vi "HostCoordinateCalibration.vi"(0 "stop_sign_queue":refnum<queue>, 4 "RetRate um/s":dbl format="%#_13g", 5 "AppRate um/s":dbl format="%#_13g", 6 "Retract um":dbl format="%#_13g", 7 "Threshold %":dbl format="%#_13g", 8 "YCalibrationEnd um":dbl format="%#_13g", 9 "XCalibrationEnd um":dbl format="%#_13g", 10 "YCalibrationOffset um":dbl format="%#_13g", 11 "XCalibrationOffset um":dbl format="%#_13g") -> (3 "img_bundle":i32[][][](array[numeric]))   [LabVIEW 2024]
uses:
  <vilib>/FPGAPlugInAG/USB-7845R OEM/niLvFpga_Open_USB-7845R OEM.vi
  <vilib>/rvi/interface/common/dynamic/niFpgaDynamicAddResources.vi
  <vilib>/Utility/error.llb/Error Cluster From Error Code.vi
  <vilib>/rvi/errors/niLvFpgaAdjustHostInterfaceError.vi
  <vilib>/FPGAPlugInAG/Dynamic/niLvFpga_Close_Dynamic.vi
  <vilib>/rvi/interface/nirviOpenFPGA/nirviOpenFPGA.xnode
  FPGA Bitfiles/hoppingsicmv2_FPGATarget_FPGAThreePointSu_uJek5trFx5s.lvbitx
  <vilib>/rvi/interface/nirviReadWriteControl/nirviReadWriteControl.xnode
  <vilib>/rvi/interface/nirviMethod/nirviMethod.xnode
  <vilib>/rvi/interface/nirviCloseFPGA/nirviCloseFPGA.xnode
  NiFpgaLv.dll
  <vilib>/rvi/interface/Simulation/niFpgaSimulationCallBeginRW.vi
  <vilib>/FPGAPlugInAG/Dynamic/niLvFpga_ReadFifo_Dynamic.vi
  <vilib>/rvi/errors/niLvFpgaMergeErrorWithErrorCode.vi
  <vilib>/FPGAPlugInAG/Dynamic/niLvFpga_WriteFifo_Dynamic.vi
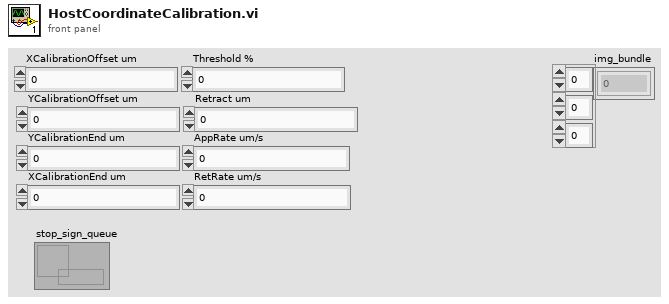
[diagram p1: front panel]
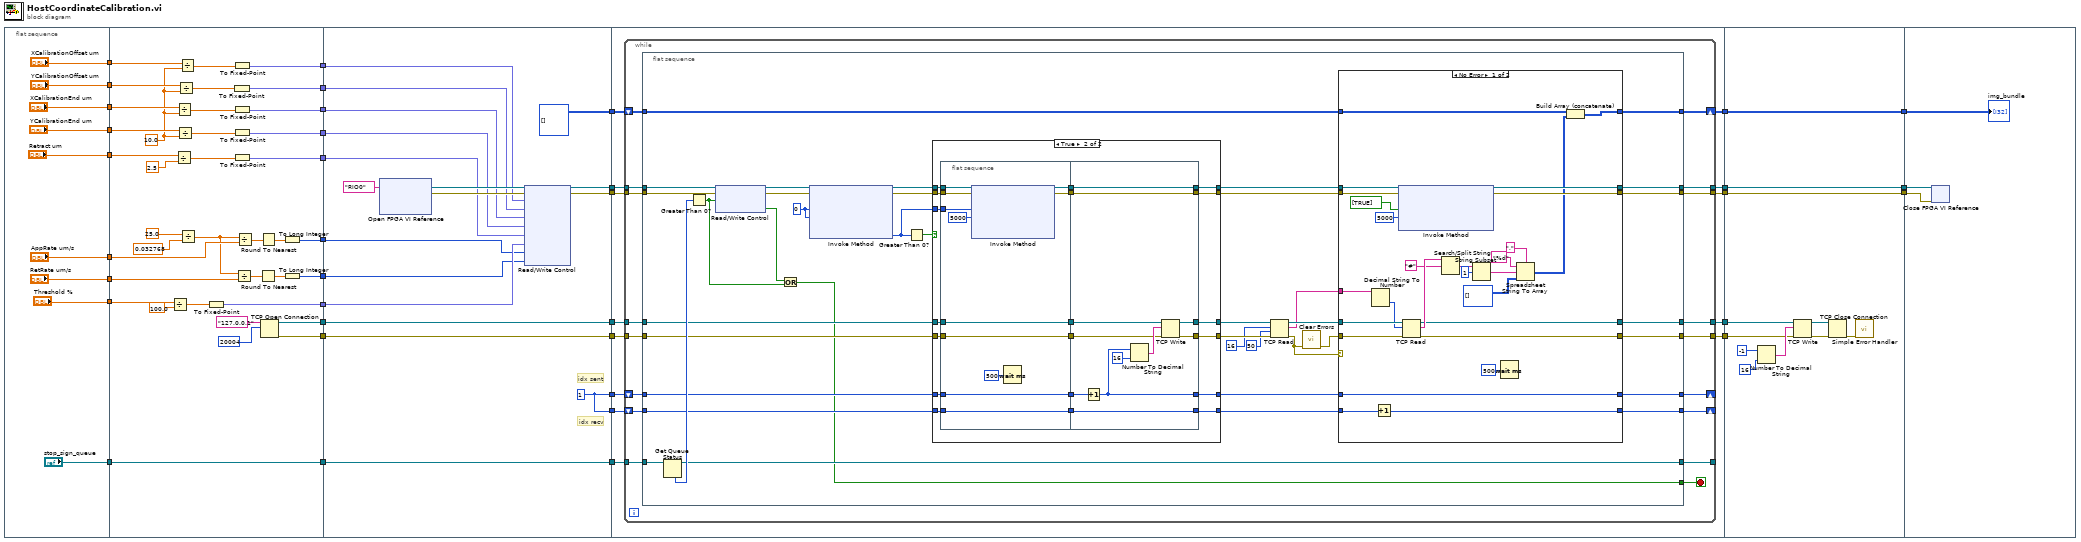
[diagram p0: block diagram]
diagram:
  n1 = flat-sequence {
    tunnel: ["Threshold %"] -> w36
    tunnel: ["AppRate um/s"] -> w35
    tunnel: ["RetRate um/s"] -> w34
    tunnel: ["Retract um"] -> w30
    tunnel: ["YCalibrationEnd um"] -> w29
    tunnel: ["XCalibrationEnd um"] -> w28
    tunnel: ["YCalibrationOffset um"] -> w27
    tunnel: ["XCalibrationOffset um"] -> w26
    tunnel: ["stop_sign_queue"] -> w16
    tunnel: w36 -> [w80]
    tunnel: w35 -> [w75]
    tunnel: w34 -> [w46]
    tunnel: [w72] -> w33
    tunnel: [w71] -> w32
    tunnel: [w70] -> w31
    tunnel: w30 -> [w69]
    tunnel: w29 -> [w67]
    tunnel: w28 -> [w66]
    tunnel: w27 -> [w62]
    tunnel: w26 -> [w61]
    tunnel: [w57] -> w25
    tunnel: [w56] -> w24
    tunnel: [w55] -> w23
    tunnel: [w54] -> w22
    tunnel: [w53] -> w21
    tunnel: [w50] -> w18
    tunnel: [w49] -> w17
    tunnel: w16 -> [w48]
    tunnel: [w48] -> w15
    tunnel: w33 -> [w89]
    tunnel: w32 -> [w88]
    tunnel: w31 -> [w90]
    tunnel: w25 -> [w95]
    tunnel: w24 -> [w94]
    tunnel: w23 -> [w93]
    tunnel: w22 -> [w92]
    tunnel: w21 -> [w91]
    tunnel: [w97] -> w20
    tunnel: [w96] -> w19
    tunnel: w18 -> [w86]
    tunnel: w17 -> [w85]
    tunnel: w15 -> [w87]
    tunnel: [w87] -> w14
    tunnel: [w86] -> w13
    tunnel: [w85] -> w12
    tunnel: [i32[][][] []] -> w11
    tunnel: [w83] -> w10
    tunnel: [w83] -> w9
    tunnel: w20 -> [w113]
    tunnel: w19 -> [w112]
    tunnel: w14 -> [w111]
    tunnel: w13 -> [w110]
    tunnel: w12 -> [w109]
    tunnel: w11 -> [w108]
    tunnel: w10 -> [w107]
    tunnel: w9 -> [w106]
    tunnel: [w105] -> w8
    tunnel: [w104] -> w6
    tunnel: [w103] -> w4
    tunnel: [w102] -> w2
    tunnel: [w101] -> w1
    tunnel: w8 -> [w261]
    tunnel: [w261] -> w7
    tunnel: w6 -> [w260]
    tunnel: [w260] -> w5
    tunnel: w4 -> [w259]
    tunnel: [w259] -> w3
    tunnel: w2 -> [w255]
    tunnel: w1 -> [w254]
    tunnel: w7 -> [w264]
    tunnel: w5 -> [w263]
    tunnel: w3 -> [w262]
    frame #0 {
    }
    frame #1 {
      w60 = 10.0
      n2 = Divide(x=w80, y=100.0) -> (x/y=w82:dbl)
      n3 = Divide(x=w69, y=2.5) -> (x/y=w65:dbl)
      n4 = Divide(x=w66, y=w60) -> (x/y=w63:dbl)
      n5 = Divide(x=w67, y=w60) -> (x/y=w64:dbl)
      n6 = Divide(x=w62, y=w60) -> (x/y=w58:dbl)
      n7 = Divide(x=w61, y=w60) -> (x/y=w59:dbl)
      n8 = Divide(x=25.0, y=0.032768) -> (x/y=w47:dbl)
      n9 = To Fixed-Point(number=w82) -> (fixed-point=w70:fxp<+/-,48,16>)  [unwired: 1 in]
      n10 = To Fixed-Point(number=w58) -> (fixed-point=w56:fxp<+/-,48,16>)  [unwired: 1 in]
      n11 = To Fixed-Point(number=w59) -> (fixed-point=w57:fxp<+/-,48,16>)  [unwired: 1 in]
      n12 = To Fixed-Point(number=w63) -> (fixed-point=w55:fxp<+/-,48,16>)  [unwired: 1 in]
      n13 = To Fixed-Point(number=w64) -> (fixed-point=w54:fxp<+/-,48,16>)  [unwired: 1 in]
      n14 = To Fixed-Point(number=w65) -> (fixed-point=w53:fxp<+/-,48,16>)  [unwired: 1 in]
      n15 = Divide(x=w47, y=w46) -> (x/y=w73:dbl)
      n16 = Divide(x=w47, y=w75) -> (x/y=w77:dbl)
      n17 = Round To Nearest(number=w73) -> (nearest integer value=w74:dbl)
      n18 = Round To Nearest(number=w77) -> (nearest integer value=w76:dbl)
      n19 = TCP Open Connection(address="127.0.0.1", remote port or service name=20004) -> (connection ID=w50:refnum<k5>, error out=w49:errorcluster)  [unwired: 3 in]
      n20 = To Long Integer(number=w74) -> (32bit integer=w71:i32)
      n21 = To Long Integer(number=w76) -> (32bit integer=w72:i32)
    }
    frame #2 {
      w83 = 1
      # "idx recv"
      # "idx sent"
      n22 = xnode "Open FPGA VI Reference"("resource name"=tag "RIO0") -> ("FPGA VI Reference Out"=w99:refnum<k20>, "error out"=w98:errorcluster)  [unwired: 1 in]
      n23 = xnode "Read/Write Control"("FPGA VI Reference In"=w99, "error in"=w98, "X_Start"=w95, "Y_Start"=w94, "X_End"=w93, "Y_End"=w92, "Retract"=w91, "Threshold"=w90, "AppRate us"=w89, "RetRate us"=w88) -> ("FPGA VI Reference Out"=w97:refnum<k20>, "error out"=w96:errorcluster)
    }
    frame #3 {
      n24 = while {
        tunnel: w113 -> [w130]
        tunnel: w112 -> [w129]
        tunnel: w111 -> [w128]
        tunnel: w110 -> [w127]
        tunnel: w109 -> [w126]
        shift-right: [w121] -> w103
        shift-left: w108 -> [w125]
        shift-right: [w120] -> _
        shift-left: w107 -> [w124]
        shift-right: [w119] -> _
        shift-left: w106 -> [w123]
        tunnel: [w122] -> _
        tunnel: [w117] -> w105
        tunnel: [w116] -> w104
        tunnel: [w115] -> w102
        tunnel: [w114] -> w101
        stop <- w118 stop-if-true
        n25 = flat-sequence {
          tunnel: w125 -> [w141]
          tunnel: w126 -> [w157]
          tunnel: w127 -> [w158]
          tunnel: w128 -> [w167]
          tunnel: w129 -> [w168]
          tunnel: w130 -> [w169]
          tunnel: w124 -> [w156]
          tunnel: w123 -> [w155]
          tunnel: [w144] -> w122
          tunnel: [w138] -> w121
          tunnel: [w137] -> w120
          tunnel: [w136] -> w119
          tunnel: [w135] -> w118
          tunnel: [w134] -> w117
          tunnel: [w133] -> w116
          tunnel: [w132] -> w115
          tunnel: [w131] -> w114
          frame #0 {
            w163 = u32 0 ("Number of Elements")
            n26 = Get Queue Status(queue=w167) -> (queue out=w144:refnum<queue>, # elements in queue=w166:i32)  [unwired: 2 in, 6 out]
            n27 = Greater Than 0?(x=w166) -> (x > 0?=w142:bool)
            n28 = xnode "Read/Write Control"("FPGA VI Reference In"=w169, "error in"=w168, "stop"=w142) -> ("FPGA VI Reference Out"=w165:refnum<k20>, "error out"=w164:errorcluster, "TargetDone?"=w143:bool)
            n29 = Or(x=w143, y=w142) -> (x .or. y?=w135:bool)
            n30 = xnode "Invoke Method"("FPGA VI Reference In"=w165, "error in"=w164, "Number of Elements"=w163, "Timeout (ms)"=w163) -> ("FPGA VI Reference Out"=w162:refnum<k20>, "error out"=w161:errorcluster, "Elements Remaining"=w159:u32)  [unwired: 1 out]
            n31 = Greater Than 0?(x=w159) -> (x > 0?=w160:bool)
            n32 = case shown="True" w160 {
              tunnel: w162 -> [w209 w228]
              tunnel: w161 -> [w208 w227]
              tunnel: w159 -> [_ w226]
              tunnel: [w209 w225] -> w146
              tunnel: [w208 w224] -> w145
              tunnel: w158 -> [w207 w223]
              tunnel: w157 -> [w206 w222]
              tunnel: w156 -> [w205 w221]
              tunnel: w155 -> [w204 w214]
              tunnel: [w207 w220] -> w154
              tunnel: [w206 w219] -> w153
              tunnel: [w205 w218] -> w140
              tunnel: [w204 w212] -> w139
              frame False {
              }
              frame True {
                n33 = flat-sequence {
                  tunnel: w228 -> [w239]
                  tunnel: w227 -> [w238]
                  tunnel: w226 -> [w237]
                  tunnel: w223 -> [w231]
                  tunnel: w222 -> [w230]
                  tunnel: w221 -> [w233]
                  tunnel: [w235] -> w217
                  tunnel: [w234] -> w216
                  tunnel: [w233] -> w215
                  tunnel: w214 -> [w232]
                  tunnel: [w232] -> w213
                  tunnel: [w231] -> w211
                  tunnel: [w230] -> w210
                  tunnel: [w244] -> w218
                  tunnel: [w245] -> w219
                  tunnel: [w246] -> w220
                  tunnel: [w249] -> w224
                  tunnel: [w250] -> w225
                  tunnel: w217 -> [w250]
                  tunnel: w216 -> [w249]
                  tunnel: w215 -> [w243]
                  tunnel: w213 -> [w242]
                  tunnel: [w242] -> w212
                  tunnel: w211 -> [w241]
                  tunnel: w210 -> [w240]
                  frame #0 {
                    n34 = xnode "Invoke Method"("FPGA VI Reference In"=w239, "error in"=w238, "Number of Elements"=w237, "Timeout (ms)"=5000) -> ("FPGA VI Reference Out"=w235:refnum<k20>, "error out"=w234:errorcluster)  [unwired: 2 out]
                    n35 = Wait (ms)(milliseconds to wait=u32 500) -> ()  [unwired: 1 out]
                  }
                  frame #1 {
                    n36 = Increment(x=w243) -> (x+1=w244:i32)
                    n37 = Number To Decimal String(number=w244, width (-)=i16 16) -> (decimal integer string=w248:string)
                    n38 = TCP Write(connection ID=w241, data in=w248, error in (no error)=w240) -> (connection ID out=w246:refnum<k5>, error out=w245:errorcluster)  [unwired: 1 in, 1 out]
                  }
                }
              }
            }
            n39 = TCP Read(connection ID=w154, bytes to read=16, error in (no error)=w153, 9:50 ("timeout ms (25000)")) -> (connection ID out=w150:refnum<k5>, data out=w147:string, error out=w148:errorcluster)  [unwired: 1 in]
            n40 = call <vilib>:"Clear Errors.vi"("error in (no error)"=w148) -> ("error out"=w149:errorcluster)  [unwired: 5 in, 1 out]
            n41 = case shown="No Error" w148 {
              tunnel: w150 -> [w189 w203]
              tunnel: w149 -> [w188 w202]
              tunnel: [w175 w203] -> w132
              tunnel: [w174 w202] -> w131
              tunnel: w147 -> [w190 _]
              tunnel: w146 -> [w196 w201]
              tunnel: w145 -> [w195 w200]
              tunnel: w141 -> [w173 w197]
              tunnel: [w192 w201] -> w134
              tunnel: [w191 w200] -> w133
              tunnel: w140 -> [w177 w199]
              tunnel: w139 -> [w178 w198]
              tunnel: [w177 w199] -> w137
              tunnel: [w176 w198] -> w136
              tunnel: [w172 w197] -> w138
              frame No Error {
                n42 = Decimal String To Number(string=w190) -> (number=w187:i32)  [unwired: 2 in, 1 out]
                n43 = Increment(x=w178) -> (x+1=w176:i32)
                n44 = xnode "Invoke Method"("FPGA VI Reference In"=w196, "error in"=w195, "Data"=bool[] [TRUE], "Timeout (ms)"=5000) -> ("FPGA VI Reference Out"=w192:refnum<k20>, "error out"=w191:errorcluster)  [unwired: 1 out]
                n45 = TCP Read(connection ID=w189, bytes to read=w187, error in (no error)=w188) -> (connection ID out=w175:refnum<k5>, data out=w186:string, error out=w174:errorcluster)  [unwired: 2 in]
                n46 = Search/Split String(string=w186, search string/char (-)="#") -> (match + rest of string=w183:string)  [unwired: 1 in, 2 out]
                n47 = String Subset(string=w183, offset (0)=1) -> (substring=w182:string)  [unwired: 1 in]
                n48 = Wait (ms)(milliseconds to wait=u32 500) -> ()  [unwired: 1 out]
                n49 = Spreadsheet String To Array(delimiter (Tab)=",", format string="%d", spreadsheet string=w182, array type (2D Dbl)=i32[][] []) -> (array=w170:i32[][])
                n50 = Build Array (concatenate)(w173, w170) -> (w172:i32[][][])
              }
              frame Error {
              }
            }
          }
        }
      }
    }
    frame #4 {
      n51 = Number To Decimal String(number=-1, width (-)=i16 16) -> (decimal integer string=w257:string)
      n52 = TCP Write(connection ID=w255, data in=w257, error in (no error)=w254) -> (connection ID out=w252:refnum<k5>, error out=w251:errorcluster)  [unwired: 1 in, 1 out]
      n53 = TCP Close Connection(connection ID=w252, error in (no error)=w251) -> (error out=w253:errorcluster)  [unwired: 1 in, 1 out]
      n54 = call <vilib>:"Simple Error Handler.vi"("error in (no error)"=w253) -> ()  [unwired: 4 in, 5 out]
    }
    frame #5 {
      n55 = xnode "Close FPGA VI Reference"("FPGA VI Reference In"=w264, "error in"=w263) -> ()  [unwired: 1 out]
      "img_bundle" <- w262
    }
  }
